vi "setForces.vi"(11 "CtrlEffArray In":fxp<+/-,25,5>[](array[numeric])=[0.0, 0.0, 0.0, 0.0, 0.0]) -> (3 "ForceArray Out":fxp<+/-,25,5>[](array[numeric]) format="%#.10g")   [LabVIEW 2020, in "CtrlEff.lvlib"]
doc: "Sets the absolute value of the force actuation value for the electrodes."
uses:
  CtrlEff.lvlib
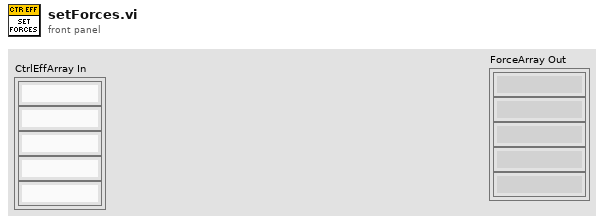
[diagram p1: front panel]
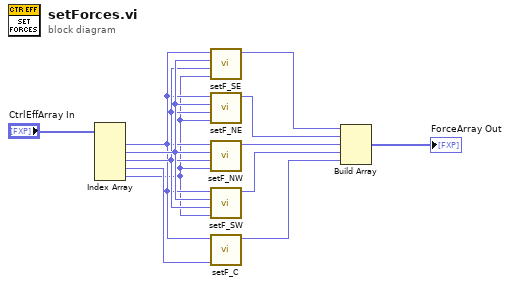
[diagram p0: block diagram]
diagram:
  n1 = Index Array(array="CtrlEffArray In") -> (element #1=w8:fxp<+/-,25,5>, element #2=w11:fxp<+/-,25,5>, element #3=w10:fxp<+/-,25,5>, element #4=w7:fxp<+/-,25,5>, element #5=w1:fxp<+/-,25,5>)  [unwired: 5 in]
  n2 = call "setF_SE.vi"("U_Bd"=w1, "U_ThY"=w10, "U_ThX"=w11, "U_Z"=w8) -> ("F_SE out"=w6:fxp<+/-,25,5>)  [unwired: 7 in]
  n3 = call "setF_NE.vi"("U_Bd"=w1, "U_ThY"=w10, "U_ThX"=w11, "U_Z"=w8) -> ("F_NE out"=w5:fxp<+/-,25,5>)  [unwired: 7 in]
  n4 = call "setF_NW.vi"("U_Bd"=w1, "U_ThY"=w10, "U_ThX"=w11, "U_Z"=w8) -> ("F_NW out"=w4:fxp<+/-,25,5>)  [unwired: 7 in]
  n5 = call "setF_SW.vi"("U_Bd"=w1, "U_ThY"=w10, "U_ThX"=w11, "U_Z"=w8) -> ("F_SW out"=w3:fxp<+/-,25,5>)  [unwired: 7 in]
  n6 = call "setF_C.vi"("U_Bow"=w7, "U_Z"=w8) -> ("F_C out"=w2:fxp<+/-,25,5>)  [unwired: 9 in]
  n7 = Build Array(w6, w5, w4, w3, w2) -> (→"ForceArray Out":fxp<+/-,25,5>[])
